vi "Read File Id.vi"(8 "error in (no error)":errorcluster, 11 "AcquireTraces in":refnum<class "AcquireTraces.lvclass">) -> (0 "error out":errorcluster, 2 "File Id":u64, 3 "AcquireTraces out":refnum<class "AcquireTraces.lvclass">)   [LabVIEW 2014, in "AcquireTraces.lvclass"]
uses:
  AcquireTraces.lvclass
  AcquireTraces.lvclass/AcquireTraces.ctl
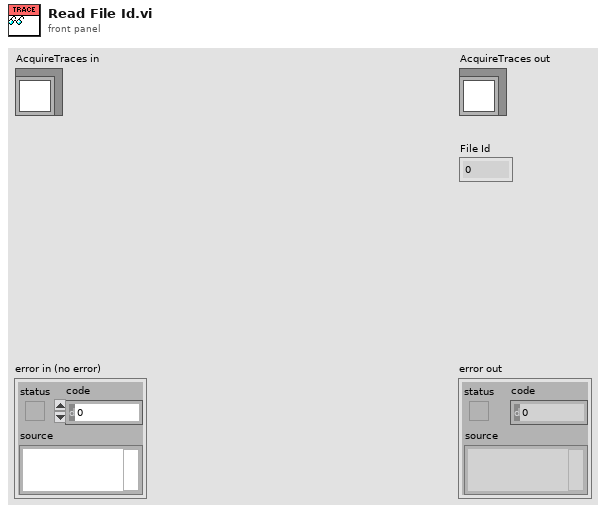
[diagram p1: front panel]
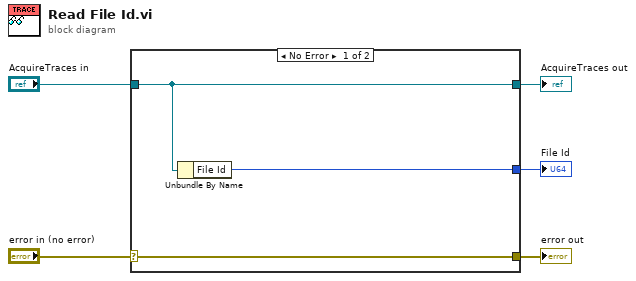
[diagram p0: block diagram]
diagram:
  n1 = case shown="No Error" "error in (no error)" {
    selector: "error in (no error)" -> [w8 w9]
    tunnel: [w8 w9] -> w4
    tunnel: [w7 w10] -> w2
    tunnel: "AcquireTraces in" -> [w7 w10]
    tunnel: [w6 _] -> w1
    frame No Error {
      n2 = Unbundle By Name(w7) -> ("File Id"=w6:u64)
    }
    frame Error {
    }
  }
  "error out" <- w4
  "AcquireTraces out" <- w2
  "File Id" <- w1
